vi "Place dots fixed.vi"(6 "Right Corner":cluster{"X":sgl, "Y":sgl}[](array[cluster]), 8 "Left Height":dbl, 9 "Left Orientation":dbl, 10 "Left Corner":cluster{"X":sgl, "Y":sgl}[](array[cluster]), 11 "Image IN":T1) -> (3 "Image OUT":T1)   [LabVIEW 2018]
uses:
  <vilib>/vision/Image Controls.llb/IMAQ Image.ctl
  Dashboard globals.vi
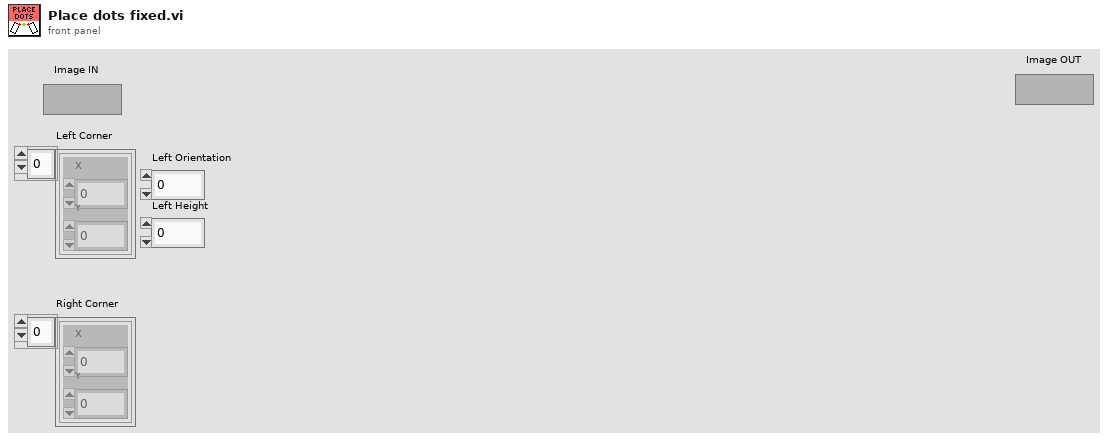
[diagram p1: front panel]
types:
  T1 = typedef "IMAQ Image.ctl" = refnum<image>
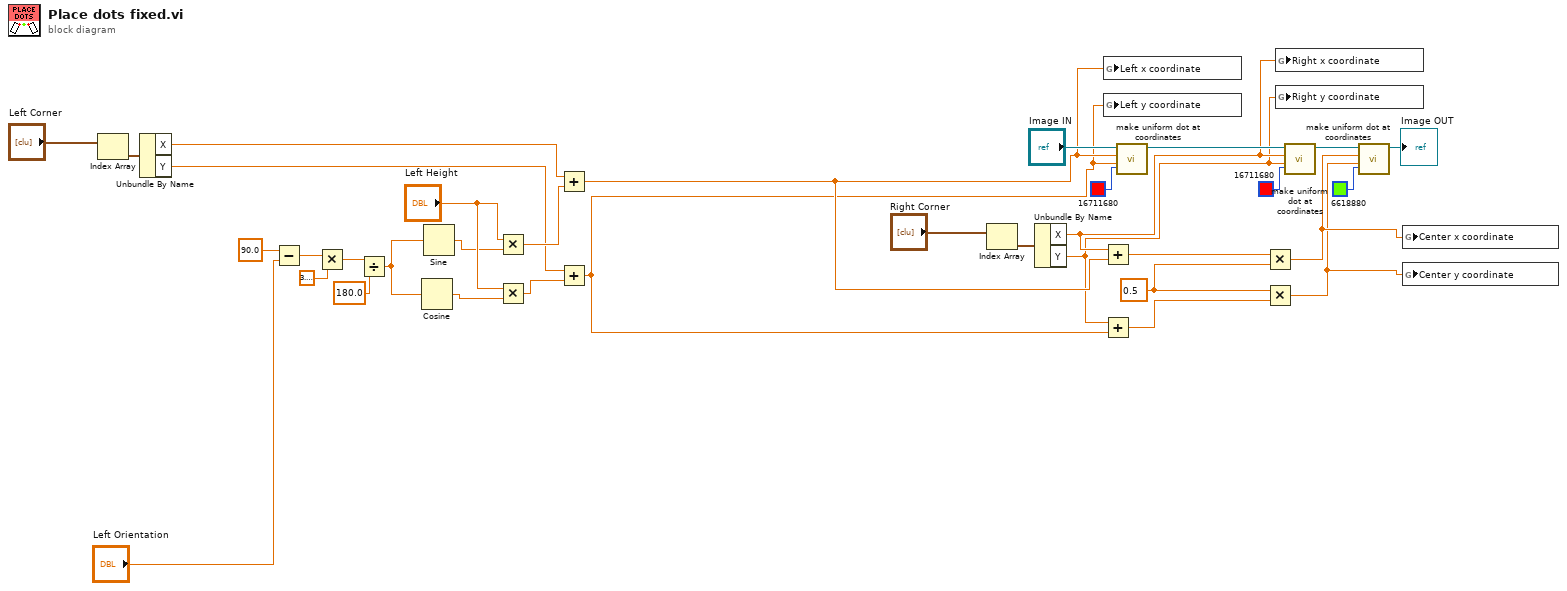
[diagram p0: block diagram]
diagram:
  w15 = 0.5 ("x")
  n1 = Index Array(array="Left Corner") -> (element=w33:cluster{"X":sgl, "Y":sgl})  [unwired: 1 in]
  n2 = Unbundle By Name(w33) -> ("X"=w19:sgl, "Y"=w18:sgl)
  n3 = Subtract(x=90.0, y="Left Orientation") -> (x-y=w29:dbl)
  n4 = Multiply(x=w29, y=3.141592653589793) -> (x*y=w27:dbl)
  n5 = Divide(x=w27, y=180.0) -> (x/y=w25:dbl)
  n6 = Cosine(x=w25) -> (cos(x)=w22:dbl)
  n7 = Sine(x=w25) -> (sin(x)=w23:dbl)
  n8 = Multiply(x="Left Height", y=w23) -> (x*y=w21:dbl)
  n9 = Multiply(x="Left Height", y=w22) -> (x*y=w20:dbl)
  n10 = Add(x=w19, y=w21) -> (x+y=w4:dbl)
  n11 = Add(x=w18, y=w20) -> (x+y=w3:dbl)
  n12 = Index Array(array="Right Corner") -> (element=w32:cluster{"X":sgl, "Y":sgl})  [unwired: 1 in]
  n13 = Unbundle By Name(w32) -> ("X"=w2:sgl, "Y"=w1:sgl)
  n14 = Add(x=w2, y=w4) -> (x+y=w16:dbl)
  n15 = Add(x=w1, y=w3) -> (x+y=w14:dbl)
  n16 = global write "Dashboard globals.vi" "Left x coordinate"(w4) -> ()
  n17 = global write "Dashboard globals.vi" "Left y coordinate"(w3) -> ()
  n18 = call "make uniform dot at coordinates.vi"("Color"=u32 16711680, "Y"=w3, "X"=w4, "Refnum in"="Image IN") -> ("Refnum out"=w12:T1)  [unwired: 7 in]
  n19 = Multiply(x=w16, y=w15) -> (x*y=w6:dbl)
  n20 = Multiply(x=w15, y=w14) -> (x*y=w5:dbl)
  n21 = global write "Dashboard globals.vi" "Right x coordinate"(w2) -> ()
  n22 = global write "Dashboard globals.vi" "Right y coordinate"(w1) -> ()
  n23 = call "make uniform dot at coordinates.vi"("Color"=u32 16711680, "Y"=w1, "X"=w2, "Refnum in"=w12) -> ("Refnum out"=w10:T1)  [unwired: 7 in]
  n24 = call "make uniform dot at coordinates.vi"("Color"=u32 6618880, "Y"=w5, "X"=w6, "Refnum in"=w10) -> ("Refnum out"=→"Image OUT":T1)  [unwired: 7 in]
  n25 = global write "Dashboard globals.vi" "Center x coordinate"(w6) -> ()
  n26 = global write "Dashboard globals.vi" "Center y coordinate"(w5) -> ()
